vi "replaceLibraryCallsScript.vi"() -> ()   [LabVIEW 2016]
uses:
  Typedefs/LibraryMemberNameReplacement.ctl
  Typedefs/LibraryDirectories.ctl
  Project/Project.lvclass
  ProjectItemFactory/ProjectItemFactory.lvclass
  C:/LSST_TS/SystemSW/ct_tools/IProjectItemFactory/IProjectItemFactory.lvclass
  Project/Project.lvclass/Project.ctl
panel:
  in  "LibraryDirectories":T1={"OldLibraryDirectory"="LibA", "NewLibraryDirectory"="LibB"}
  in  "Library Member Name Replacement":T2={"String To Replace in VI names"="A", "String To Replace in Control names"="", "New String in VI names"="B", "New String in Control names"=""}
  in  "Libraries":T3={"OldLibrary"="LibA.lvlib", "NewLibrary"="LibB.lvlib"}
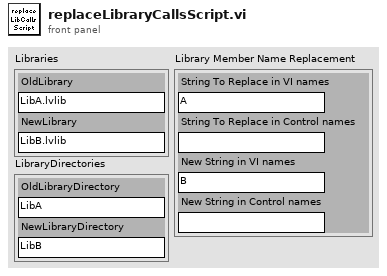
[diagram p1: front panel]
types:
  T1 = typedef "LibraryDirectories.ctl" = cluster{"OldLibraryDirectory":string, "NewLibraryDirectory":string}
  T2 = typedef "LibraryMemberNameReplacement.ctl" = cluster{"String To Replace in VI names":string, "String To Replace in Control names":string, "New String in VI names":string, "New String in Control names":string}
  T3 = cluster{"OldLibrary":string, "NewLibrary":string}
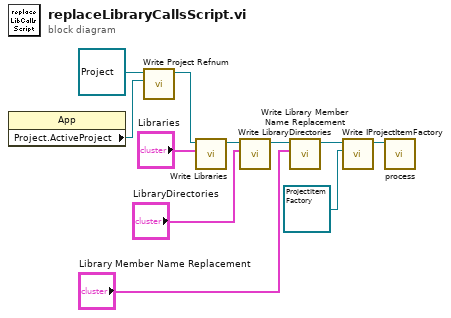
[diagram p0: block diagram]
diagram:
  n1 = property class="App"() -> ("Project.ActiveProject"=w10:refnum<vi>)  [unwired: 2 in, 2 out]
  n2 = call "Write Project Refnum.vi"("Project Refnum"=w10, "Project in"=refnum<class "Project.lvclass"> refnum ("Project.lvclass")) -> ("Project out"=w9:refnum<class "Project.lvclass">)  [unwired: 9 in]
  n3 = call "Write Libraries.vi"("Libraries"="Libraries", "Project in"=w9) -> ("Project out"=w3:refnum<class "Project.lvclass">)  [unwired: 9 in]
  n4 = call "Write LibraryDirectories.vi"("LibraryDirectories"="LibraryDirectories", "Project in"=w3) -> ("Project out"=w2:refnum<class "Project.lvclass">)  [unwired: 9 in]
  n5 = call "Write Library Member Name Replacement.vi"("Library Member Name Replacement"="Library Member Name Replacement", "Project in"=w2) -> ("Project out"=w5:refnum<class "Project.lvclass">)  [unwired: 9 in]
  n6 = call "Write IProjectItemFactory.vi"("IProjectItemFactory"=refnum<class "ProjectItemFactory.lvclass"> refnum ("ProjectItemFactory.lvclass"), "Project in"=w5) -> ("Project out"=w6:refnum<class "Project.lvclass">)  [unwired: 9 in]
  n7 = call "process.vi"("Project in"=w6) -> ()  [unwired: 9 in, 2 out]
